vi "ASDA-A2_Motor Stop Mode.vi"(8 "error in":errorcluster, 10 "Motor Stop Mode":T1(ring), 11 "Buffer Data In":T2) -> (0 "error out":errorcluster, 3 "Buffer Data Out":T2)   [LabVIEW 2016]
uses:
  Data Def/ASDA-A2_Buffer Data.ctl
  Data Def/ASDA-A2_Write Register Data.ctl
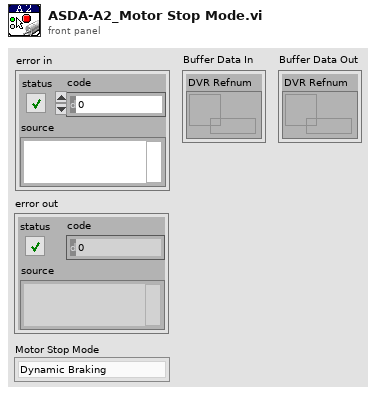
[diagram p1: front panel]
types:
  T1 = enum16{"Dynamic Braking", "Free Run", "Dynamic braking+Free Run"}
  T2 = typedef "ASDA-A2_Buffer Data.ctl" = cluster{"DVR Refnum":refnum<data-value>}
  T3 = typedef "ASDA-A2_Write Register Data.ctl" = cluster{"Address":u16, "Max Value":u32, "Min Value":u32, "Value":u32, "Type":enum16{"16 Bits", "32 Bits"}, "Page":string, "Description":string}
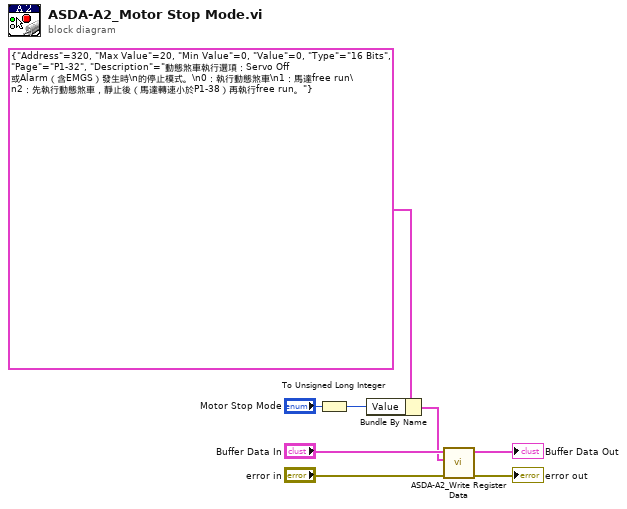
[diagram p0: block diagram]
diagram:
  n1 = To Unsigned Long Integer(number="Motor Stop Mode") -> (unsigned 32bit integer=w2:u32)
  n2 = Bundle By Name(cluster=T3 {"Address"=320, "Max Value"=20, "Min Value"=0, "Value"=0, "Type"=enum."16 Bits", "Page"="P1-32", "Description"="動態煞車執行選項：Servo Off 或Alarm（含EMGS）發生時\n的停止模式。\n0：執行動態煞車\n1：馬達free run\n2：先執行動態煞車，靜止後（馬達轉速小於P1-38）再執行free run。"} ("Write Register Data"), "Value"=w2) -> (w3:T3)
  n3 = call "ASDA-A2_Write Register Data.vi"("error in"="error in", "Write Register Data"=w3, "Buffer Data In"="Buffer Data In") -> ("error out"=→"error out":errorcluster, "Buffer Data Out"=→"Buffer Data Out":T2)  [unwired: 7 in]
